vi "SaveInfo.vi"(0 "object in":refnum<class "TDMSLogger.lvclass">, 1 "NoOfFrequencies":i32, 2 "NumberOfXPositions":i32, 3 "NumberOfYPositions":i32, 5 "error in (no error)":errorcluster, 6 "Meander?":bool=TRUE, 7 "NoOfAmplitudes":i32) -> (14 "object out":refnum<class "TDMSLogger.lvclass">, 19 "error out":errorcluster)   [LabVIEW 2023, in "TDMSLogger.lvclass"]
uses:
  TDMSLogger.lvclass
  TDMSLogger.lvclass/TDMSLogger.ctl
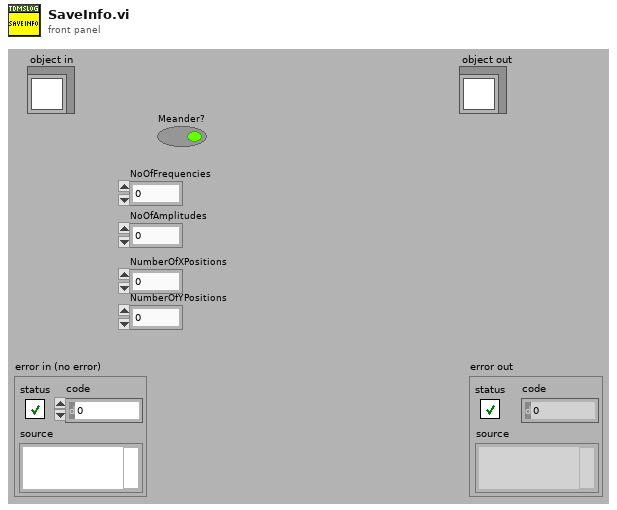
[diagram p1: front panel]
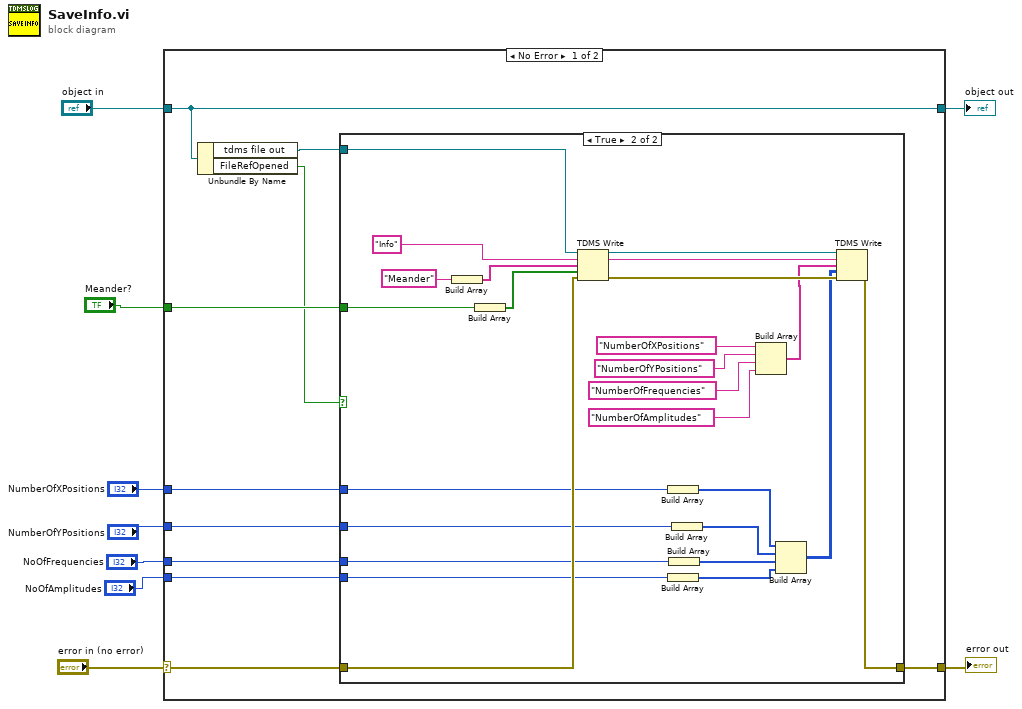
[diagram p0: block diagram]
diagram:
  n1 = case shown="No Error" "error in (no error)" {
    selector: "error in (no error)" -> [w17 w47]
    tunnel: [w18 w47] -> w8
    tunnel: [w19 w46] -> w6
    tunnel: "object in" -> [w19 w46]
    tunnel: "NumberOfXPositions" -> [w14 _]
    tunnel: "NumberOfYPositions" -> [w13 _]
    tunnel: "NoOfFrequencies" -> [w12 _]
    tunnel: "Meander?" -> [w15 _]
    tunnel: "NoOfAmplitudes" -> [w11 _]
    frame No Error {
      n2 = Unbundle By Name(w19) -> ("tdms file out"=w16:refnum<k34>, "FileRefOpened"=w10:bool)
      n3 = case shown="True" w10 {
        tunnel: [w20 w45] -> w18
        tunnel: w17 -> [w20 w40]
        tunnel: w16 -> [_ w35]
        tunnel: w15 -> [_ w31]
        tunnel: w14 -> [_ w28]
        tunnel: w13 -> [_ w26]
        tunnel: w12 -> [_ w24]
        tunnel: w11 -> [_ w22]
        frame False {
        }
        frame True {
          n4 = Build Array("Meander" ("group name in (Untitled)")) -> (w37:string[])
          n5 = Build Array(w31) -> (w36:bool[])
          n6 = TDMS Write(0:w35, 5:"Info" ("group name in (Untitled)"), 7:w37, 9:w36, 11:w40) -> (4:w41:refnum<k34>, 6:w33:string, 15:w39:errorcluster)  [unwired: 1 in, 1 out]
          n7 = Build Array(w28) -> (w29:i32[])
          n8 = Build Array(w22) -> (w21:i32[])
          n9 = Build Array(w24) -> (w25:i32[])
          n10 = Build Array(w26) -> (w27:i32[])
          n11 = Build Array("NumberOfXPositions" ("group name in (Untitled)"), "NumberOfYPositions" ("group name in (Untitled)"), "NumberOfFrequencies" ("group name in (Untitled)"), "NumberOfAmplitudes" ("group name in (Untitled)")) -> (w32:string[])
          n12 = Build Array(w29, w27, w25, w21) -> (w30:i32[][])
          n13 = TDMS Write(0:w41, 5:w33, 7:w32, 9:w30, 11:w39) -> (15:w45:errorcluster)  [unwired: 1 in, 3 out]
        }
      }
    }
    frame Error {
    }
  }
  "error out" <- w8
  "object out" <- w6
